vi "EPTxRTadd_ontest4.vi"(11 "OpWin_Setting":T4={"EPTxAAPControl_1str"={"Enable"=FALSE, "Rising_[DBTDC]"=12.0, "Falling_[DBTDC]"=-12.0}, "EPTxAAPControl_2str"={"Enable"=FALSE, "Rising_[DBTDC]"=12.0, "Falling_[DBTDC]"=-12.0}, "EPTxAAPControl_3str"={"Enable"=FALSE, "Rising_[DBTDC]"=12.0, "Falling_[DBTDC]"=-12.0}, "EPTxAAPControl_4str"={"Enable"=FALSE, "Rising_[DBTDC]"=12.0, "Falling_[DBTDC]"=-12.0}, "EPTxAAPControl_5str"={"Enable"=FALSE, "Rising_[DBTDC]"=12.0, "Falling_[DBTDC]"=-12.0}, "EPTxAAPControl_6str"={"Enable"=FALSE, "Rising_[DBTDC]"=12.0, "Falling_[DBTDC]"=-12.0}} caption="簇") -> (3 "EPTxAAPControl_rtOpWin":T2 caption="簇")   [LabVIEW 2020]
uses:
  <vilib>/Powertrain Controls/Device Drivers/Engine Position Tracking/EPTx/RevA/RT/Controls/EPTxAAPControl.ctl
  <vilib>/Powertrain Controls/Device Drivers/Engine Position Tracking/EPTx/RevA/FPGA/Controls/EPTxAAPControl.ctl
  <vilib>/Powertrain Controls/Device Drivers/Engine Position Tracking/EPTx/RevA/RT/EPTx - RevA - RT.lvlib
  <vilib>/Powertrain Controls/Device Drivers/Engine Position Tracking/EPTx/RevA/FPGA/EPTx - RevA - FPGA.lvlib
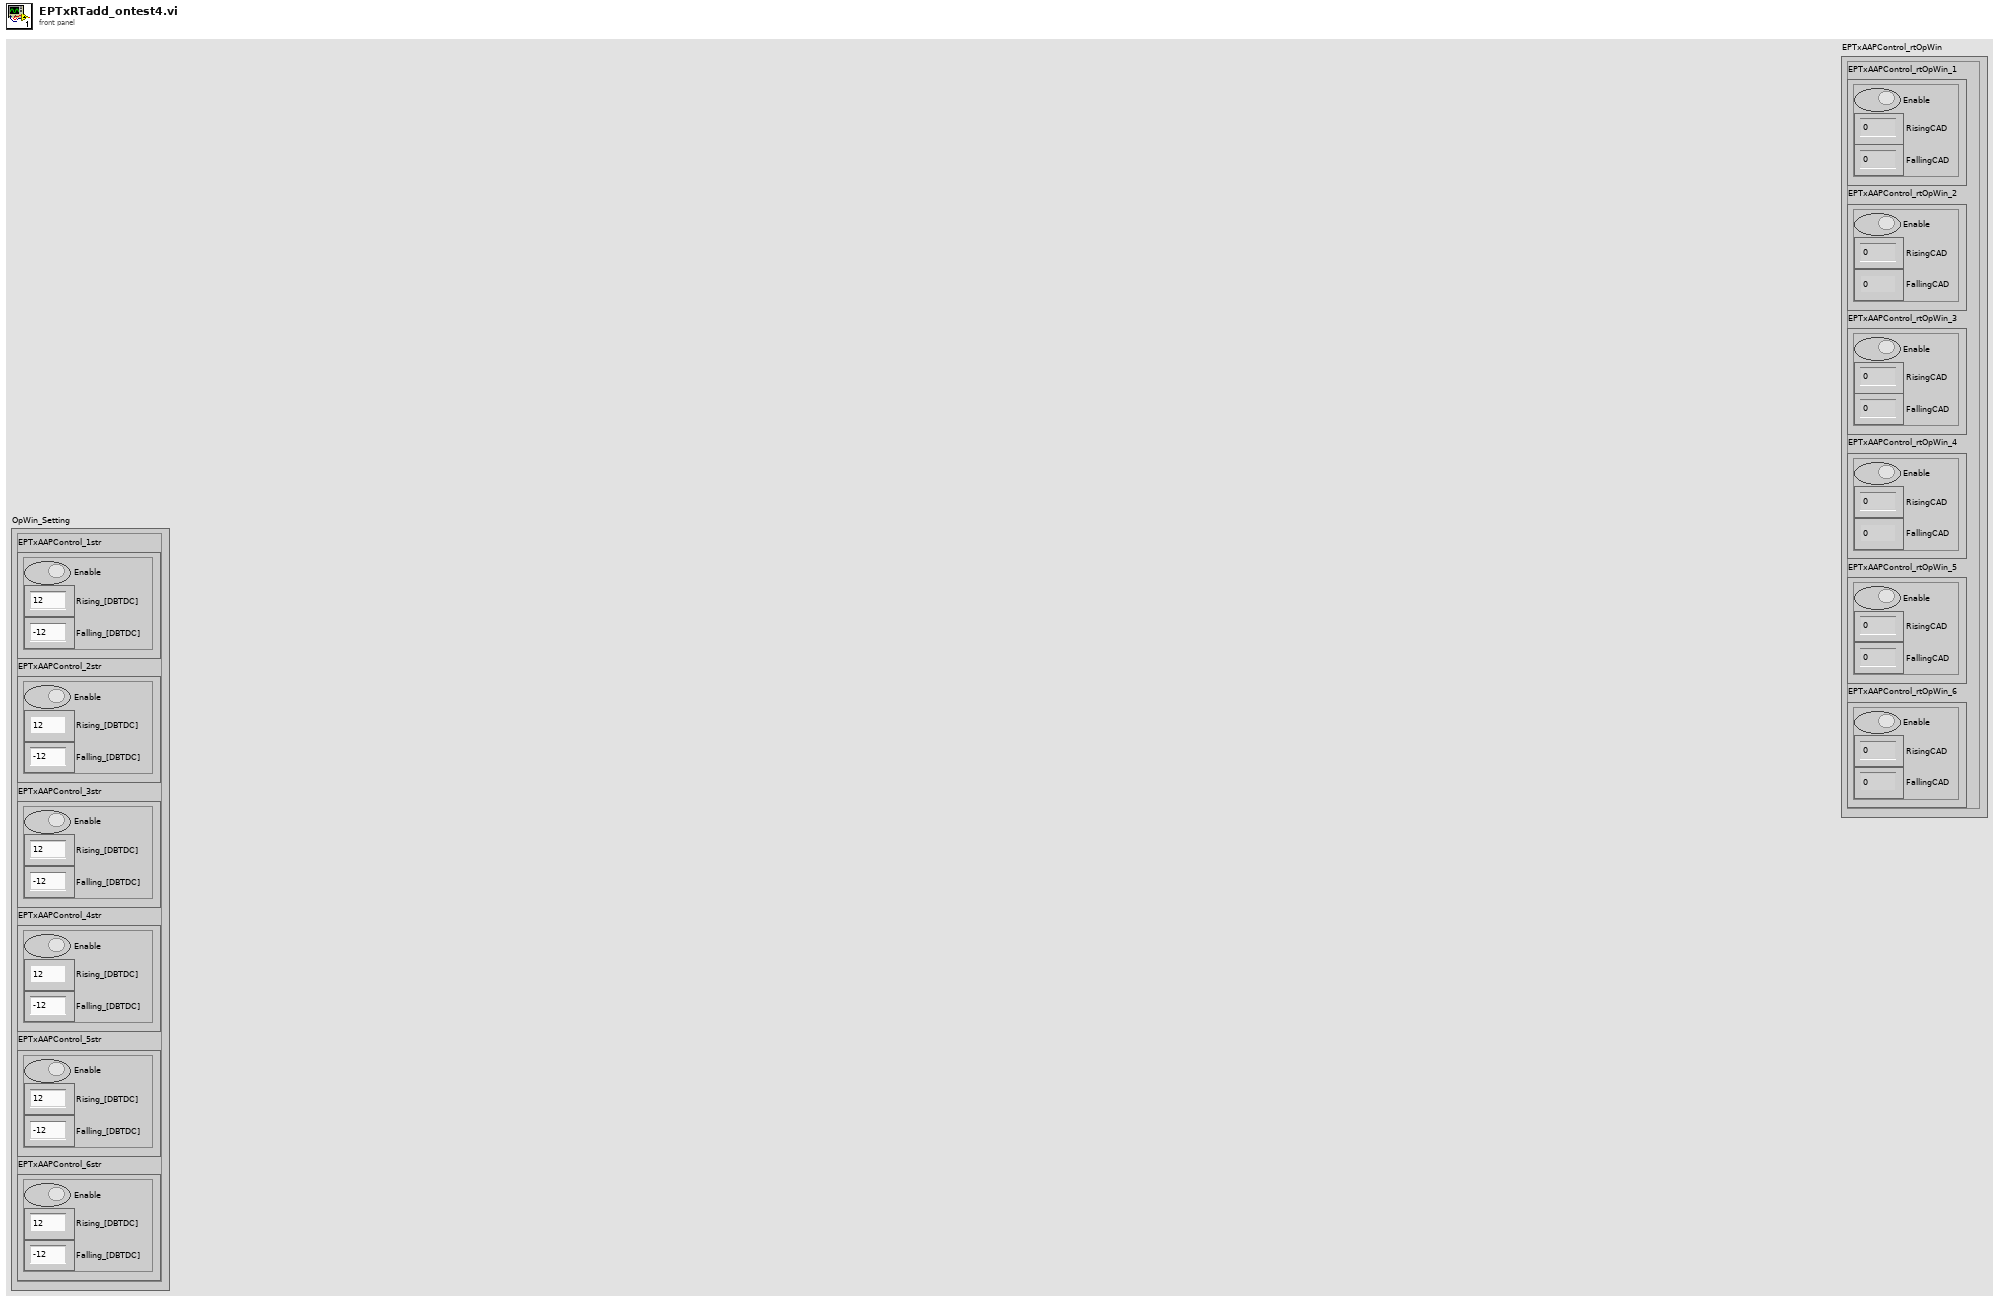
[diagram p1: front panel]
types:
  T1 = typedef "EPTx - RevA - FPGA.lvlib/EPTxAAPControl.ctl" = cluster{"Enable":bool, "RisingCAD":fxp<+,18,11>, "FallingCAD":fxp<+,18,11>}
  T2 = cluster{"EPTxAAPControl_rtOpWin_1":T1, "EPTxAAPControl_rtOpWin_2":T1, "EPTxAAPControl_rtOpWin_3":T1, "EPTxAAPControl_rtOpWin_4":T1, "EPTxAAPControl_rtOpWin_5":T1, "EPTxAAPControl_rtOpWin_6":T1}
  T3 = typedef "EPTx - RevA - RT.lvlib/EPTxAAPControl.ctl" = cluster{"Enable":bool, "Rising_[DBTDC]":sgl, "Falling_[DBTDC]":sgl}
  T4 = cluster{"EPTxAAPControl_1str":T3, "EPTxAAPControl_2str":T3, "EPTxAAPControl_3str":T3, "EPTxAAPControl_4str":T3, "EPTxAAPControl_5str":T3, "EPTxAAPControl_6str":T3}
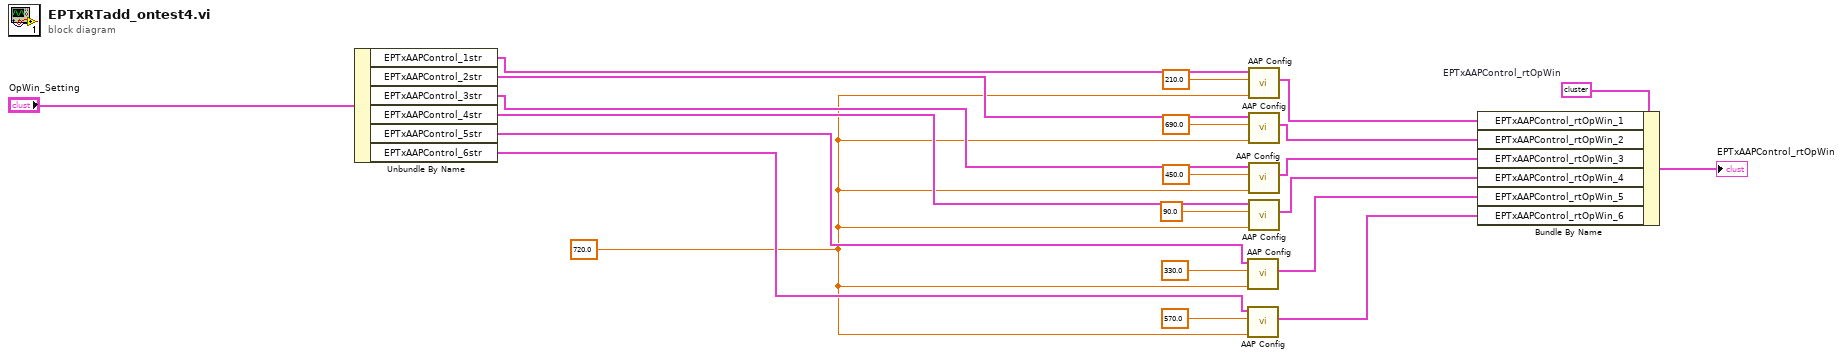
[diagram p0: block diagram]
diagram:
  w1 = sgl 720.0 ("Max CAD")
  w18 = T2 {"EPTxAAPControl_rtOpWin_1"={"Enable"=FALSE, "RisingCAD"=0.0, "FallingCAD"=0.0}, "EPTxAAPControl_rtOpWin_2"={"Enable"=FALSE, "RisingCAD"=0.0, "FallingCAD"=0.0}, "EPTxAAPControl_rtOpWin_3"={"Enable"=FALSE, "RisingCAD"=0.0, "FallingCAD"=0.0}, "EPTxAAPControl_rtOpWin_4"={"Enable"=FALSE, "RisingCAD"=0.0, "FallingCAD"=0.0}, "EPTxAAPControl_rtOpWin_5"={"Enable"=FALSE, "RisingCAD"=0.0, "FallingCAD"=0.0}, "EPTxAAPControl_rtOpWin_6"={"Enable"=FALSE, "RisingCAD"=0.0, "FallingCAD"=0.0}}  # EPTxAAPControl_rtOpWin
  n1 = Unbundle By Name("OpWin_Setting") -> ("EPTxAAPControl_1str"=w6:T3, "EPTxAAPControl_2str"=w21:T3, "EPTxAAPControl_3str"=w20:T3, "EPTxAAPControl_4str"=w19:T3, "EPTxAAPControl_5str"=w5:T3, "EPTxAAPControl_6str"=w4:T3)
  n2 = call <vilib>:"AAP Config.vi"("Max CAD"=w1, "Cylinder TDC [Absolute CAD]"=sgl 330.0, "EPTxAAPControl"=w5) -> ("EPTxAAPControl"=w3:T1)  [unwired: 8 in]
  n3 = call <vilib>:"AAP Config.vi"("Max CAD"=w1, "Cylinder TDC [Absolute CAD]"=sgl 570.0, "EPTxAAPControl"=w4) -> ("EPTxAAPControl"=w2:T1)  [unwired: 8 in]
  n4 = call <vilib>:"AAP Config.vi"("Max CAD"=w1, "Cylinder TDC [Absolute CAD]"=sgl 210.0, "EPTxAAPControl"=w6) -> ("EPTxAAPControl"=w16:T1)  [unwired: 8 in]
  n5 = call <vilib>:"AAP Config.vi"("Max CAD"=w1, "Cylinder TDC [Absolute CAD]"=sgl 690.0, "EPTxAAPControl"=w21) -> ("EPTxAAPControl"=w15:T1)  [unwired: 8 in]
  n6 = call <vilib>:"AAP Config.vi"("Max CAD"=w1, "Cylinder TDC [Absolute CAD]"=sgl 450.0, "EPTxAAPControl"=w20) -> ("EPTxAAPControl"=w14:T1)  [unwired: 8 in]
  n7 = call <vilib>:"AAP Config.vi"("Max CAD"=w1, "Cylinder TDC [Absolute CAD]"=sgl 90.0, "EPTxAAPControl"=w19) -> ("EPTxAAPControl"=w13:T1)  [unwired: 8 in]
  n8 = Bundle By Name(cluster=w18, "EPTxAAPControl_rtOpWin_1"=w16, "EPTxAAPControl_rtOpWin_2"=w15, "EPTxAAPControl_rtOpWin_3"=w14, "EPTxAAPControl_rtOpWin_4"=w13, "EPTxAAPControl_rtOpWin_5"=w3, "EPTxAAPControl_rtOpWin_6"=w2) -> (→"EPTxAAPControl_rtOpWin":T2)
